vi "SetTrigger.vi"(4 "Start Trigger":i16(ring) items=["Only at the start of the sequence"=0, "On each bank"=256, "On each curve in the bank"=768], 6 "Ext. Trigger Condition":i16(ring) items=["None", "Falling Edge", "Rising Edge"], 7 "Master":bool, 8 "Error In":errorcluster, 10 "Module No":i16, 11 "DLL Path":path) -> (0 "Error Out":errorcluster, 2 "Module No":i16, 3 "DLL Path":path)   [LabVIEW 2017]
doc: "This VI is a wrapper for SPC_set_parameter.vi with the 'SPC parameter ID' set to 'External Trigger Condition'. The flag values are calculated for convenience.\n\ninfo@becker-hickl.com"
uses:
  SPC_Controls/par_id.ctl
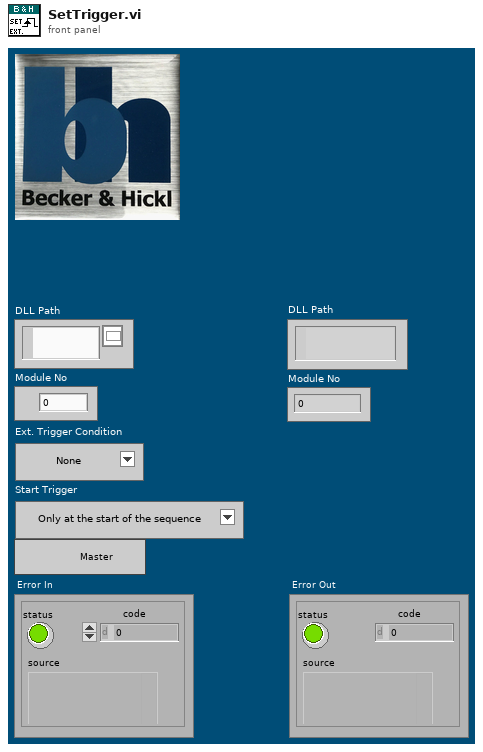
[diagram p1: front panel]
types:
  T1 = typedef "par_id.ctl" = i16
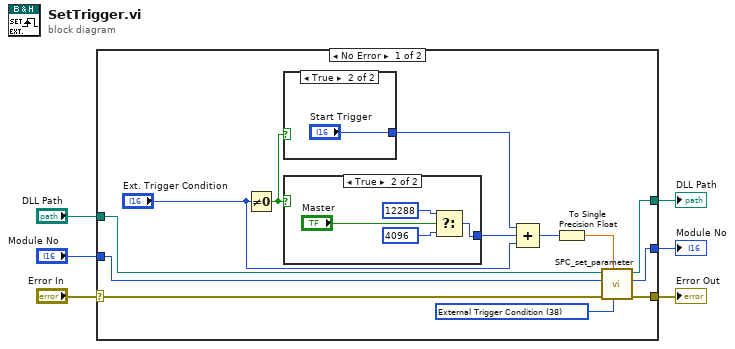
[diagram p0: block diagram]
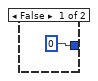
[diagram p2: hidden frame]
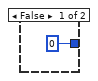
[diagram p3: hidden frame]
diagram:
  n1 = case shown="No Error" "Error In" {
    selector: "Error In" -> [w19 w27]
    tunnel: [w18 w27] -> w5
    tunnel: "Module No" -> [w17 w28]
    tunnel: [w16 w28] -> w3
    tunnel: "DLL Path" -> [w15 w29]
    tunnel: [w14 w29] -> w1
    frame No Error {
      w7 = T1 38 items=["CFD Limit Low", "CFD Limit High", "CFD Zero Cross Level", "CFD Holdoff", "SYNC Zero Cross Level", "SYNC Freq Divider", "SYNC Holdoff", "SYNC Threshold", "TAC Range", "TAC Gain", "TAC Offset", "TAC Limit Low", "TAC Limit High", "ADC Resolution", "External Latch Delay", "Collect Time", "Display Time", "Repeat Time", "Stop On Time", "Stop On Overflow", "Dither Range", "Count Increment", "Memory Bank", "Dead Time Compensation", "Scan Control", "Routing Mode", "TAC Enable Hold", "Operation Mode", "Scan Size X", "Scan Size Y", "Scan Routing X Bits", "Scan Routing Y Bits", "Scan Polarity", "Scan Flyback", "Scan Borders", "Pixel Time", "Pixel Clock Source", "Scan Line Compression", "External Trigger Condition", "External Pixel Clock Divider", "Rate Counting Time", "Macro Time Clock", "ADD Signal Source", "ADC Zoom", "XY Gain", "Image Size X", "Image Size Y", "Image Routing X Bits", "Image Routing Y Bits", "Master Clock", "ADC Sample Delay", "Detector Type", "X Axis Type", "Channel Enable", "Channel Slope", "Channel Spec_no"] ("SPC parameter ID")
      n2 = Not Equal To 0?(x="Ext. Trigger Condition") -> (x != 0?=w11:bool)
      n3 = case shown="True" w11 {
        tunnel: [i16 0 "Start Trigger"] -> w10
        frame False {
        }
        frame True {
        }
      }
      n4 = case shown="True" w11 {
        tunnel: [i16 0 w23] -> w12
        frame False {
        }
        frame True {
          n5 = Select(t=i16 12288, s="Master", f=i16 4096) -> (s? t:f=w23:i16)
        }
      }
      n6 = Compound Arithmetic op=ADD(w10, w12, "Ext. Trigger Condition") -> (w9:i16)
      n7 = To Single Precision Float(number=w9) -> (single precision float=w8:sgl)
      n8 = call "SPC_set_parameter.vi"("SPC parameter ID"=w7, "Parameter Value"=w8, "Error In"=w19, "Module no"=w17, "DLL Path"=w15) -> ("Error Out"=w18:errorcluster, "Module no"=w16:i16, "DLL Path"=w14:path)  [unwired: 3 in, 1 out]
    }
    frame Error {
    }
  }
  "Error Out" <- w5
  "Module No" <- w3
  "DLL Path" <- w1
